vi "Create RSA Key.vi"(5 "Key Length (2048)":i32=2048, 6 "Machine Key?":bool, 7 "Crypto Provider":T1, 8 "error in (no error)":errorcluster, 9 "Export Policy (allow export)":i32(ring)=1 items=["None"=0, "AllowExport"=1, "AllowPlaintextExport"=2, "AllowArchiving"=4, "AllowPlaintextArchiving"=8], 10 "Key Usage (all usages)":i32(ring)=16777215 items=["None"=0, "Decryption"=1, "Signing"=2, "KeyAgreement"=4, "AllUsages"=16777215], 11 "Key Name":string) -> (0 "error out":errorcluster, 3 "CngKey out":refnum<k24>)   [LabVIEW 2021, in "dotNET Crypto Key Management.lvlib"]
uses:
  dotNET Crypto Key Management.lvlib
  System.Core
  CNG Provider Type.ctl
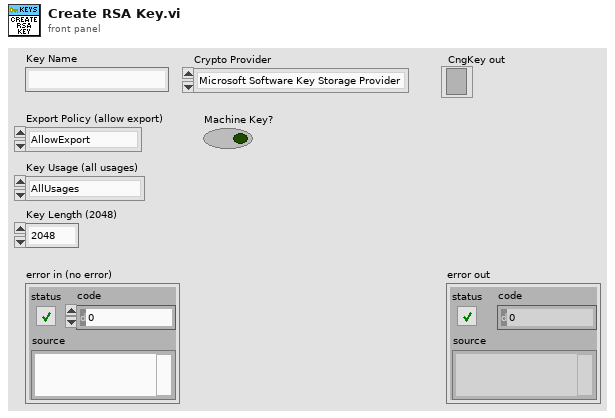
[diagram p1: front panel]
types:
  T1 = typedef "dotNET Crypto Key Management.lvlib/CNG Provider Type.ctl" = enum16{"Microsoft Software Key Storage Provider", "Microsoft Platform Crypto Provider"}
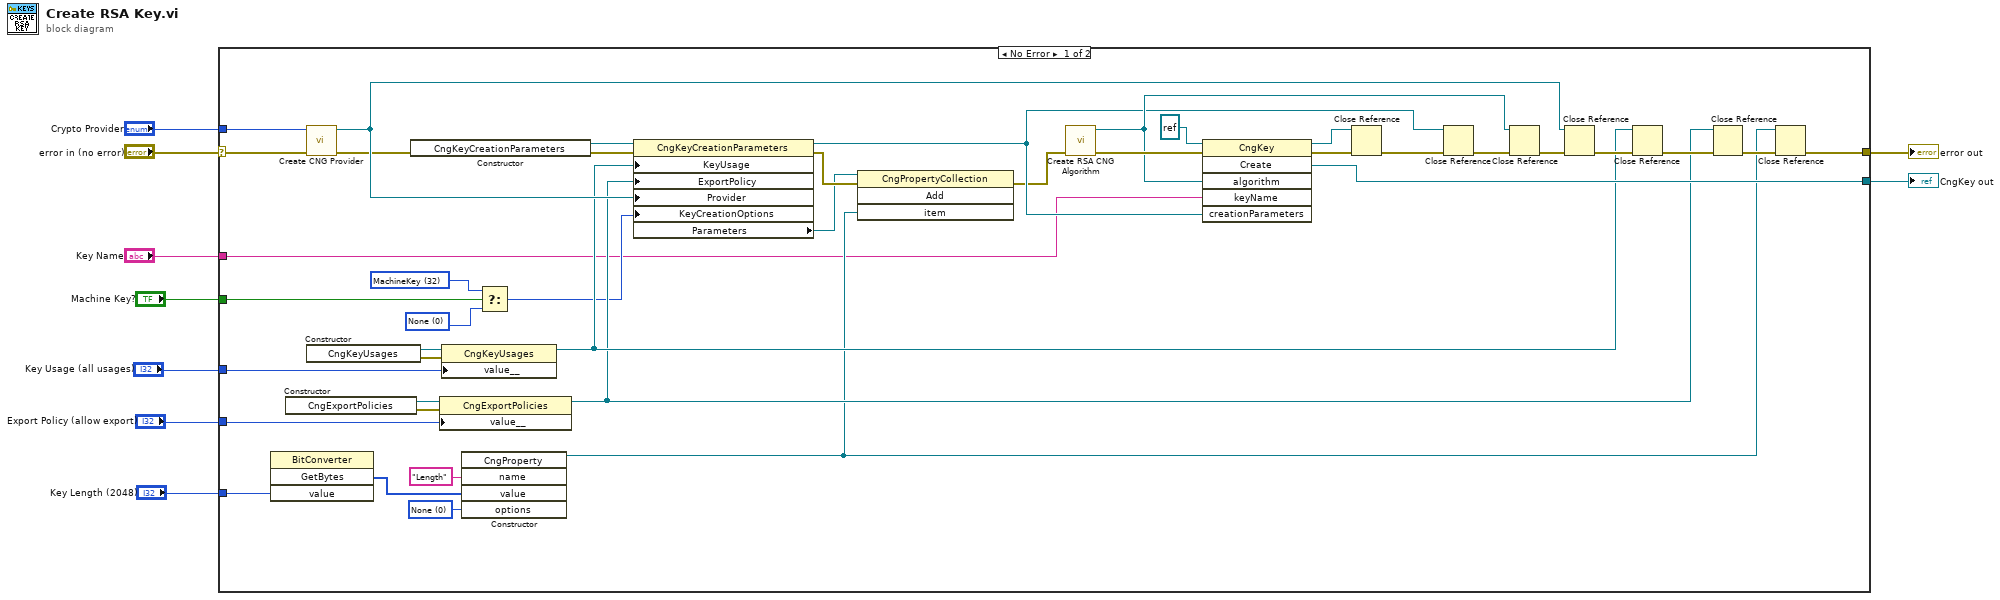
[diagram p0: block diagram]
diagram:
  n1 = case shown="No Error" "error in (no error)" {
    selector: "error in (no error)" -> [w37 w51]
    tunnel: [w49 _] -> w9
    tunnel: "Key Name" -> [w10 _]
    tunnel: "Key Usage (all usages)" -> [w43 _]
    tunnel: "Export Policy (allow export)" -> [w40 _]
    tunnel: "Crypto Provider" -> [w36 _]
    tunnel: [w14 w51] -> w3
    tunnel: "Machine Key?" -> [w22 _]
    tunnel: "Key Length (2048)" -> [w12 _]
    frame No Error {
      w16 = 0 items=["None"=0, "CustomProperty"=1073741824, "Persist"=-2147483648] ("options")
      w23 = 0 items=["None"=0, "MachineKey"=32, "OverwriteExistingKey"=128] ("MachineKey")
      w24 = 32 items=["None"=0, "MachineKey"=32, "OverwriteExistingKey"=128] ("MachineKey")
      n2 = invoke class="BitConverter" method="GetBytes"("value"=w12) -> ("GetBytes"=w11:u8[])  [unwired: 3 in, 3 out]
      n3 = constructor class="CngExportPolicies"() -> (reference out=w41:refnum<k24>, error out=w42:errorcluster)  [unwired: 3 in, 1 out]
      n4 = call "Create CNG Provider.vi"("error in (no error)"=w37, "Crypto Provider"=w36) -> ("error out"=w29:errorcluster, "CngProvider"=w33:refnum<k24>)  [unwired: 8 in]
      n5 = constructor class="CngKeyUsages"() -> (reference out=w44:refnum<k24>, error out=w45:errorcluster)  [unwired: 3 in, 1 out]
      n6 = constructor class="CngKeyCreationParameters"(error in=w29) -> (reference out=w46:refnum<k24>, error out=w39:errorcluster)  [unwired: 2 in, 1 out]
      n7 = property class="CngExportPolicies"(reference=w41, error in=w42, "value__"=w40) -> (reference out=w25:refnum<k24>)  [unwired: 1 out]
      n8 = property class="CngKeyUsages"(reference=w44, error in=w45, "value__"=w43) -> (reference out=w26:refnum<k24>)  [unwired: 1 out]
      n9 = constructor class="CngProperty"("name"="Length", "value"=w11, "options"=w16) -> (reference out=w13:refnum<k24>)  [unwired: 3 in, 5 out]
      n10 = Select(t=w24, s=w22, f=w23) -> (s? t:f=w21:i32)
      n11 = property class="CngKeyCreationParameters"(reference=w46, error in=w39, "KeyUsage"=w26, "ExportPolicy"=w25, "Provider"=w33, "KeyCreationOptions"=w21) -> (reference out=w30:refnum<k24>, error out=w20:errorcluster, "Parameters"=w19:refnum<k24>)
      n12 = invoke class="CngPropertyCollection" method="Add"(reference=w19, error in=w20, "item"=w13) -> (error out=w18:errorcluster)  [unwired: 1 in, 3 out]
      n13 = call "Create RSA CNG Algorithm.vi"("error in (no error)"=w18) -> ("error out"=w38:errorcluster, "RSA Cng Algorithm"=w35:refnum<k24>)  [unwired: 9 in]
      n14 = invoke class="CngKey" method="Create"(reference=refnum<k24> refnum, error in=w38, "algorithm"=w35, "keyName"=w10, "creationParameters"=w30) -> (reference out=w50:refnum<k24>, error out=w48:errorcluster, "Create"=w49:refnum<k24>)  [unwired: 1 in, 3 out]
      n15 = Close Reference(reference=w50, error in (no error)=w48) -> (error out=w32:errorcluster)
      n16 = Close Reference(reference=w30, error in (no error)=w32) -> (error out=w31:errorcluster)
      n17 = Close Reference(reference=w35, error in (no error)=w31) -> (error out=w34:errorcluster)
      n18 = Close Reference(reference=w33, error in (no error)=w34) -> (error out=w28:errorcluster)
      n19 = Close Reference(reference=w26, error in (no error)=w28) -> (error out=w27:errorcluster)
      n20 = Close Reference(reference=w25, error in (no error)=w27) -> (error out=w15:errorcluster)
      n21 = Close Reference(reference=w13, error in (no error)=w15) -> (error out=w14:errorcluster)
    }
    frame Error {
    }
  }
  "error out" <- w3
  "CngKey out" <- w9
